vi "ProcAndStates.vi"(0 "spreadsheet string":string=" Инициализация\r\nНачало\r\nВосстановлениеУправления\r\nНачалоРаботы\r\n ОстановВсехПроцессовИстартПроцИнициализация\r\nНачало\r\n КонтрольДостоверности\r\nНачало\r\nОстановПроцессов\r\nСообК_ГУИ_НЕТ_ДОСТОВЕРНОСТИ\r\nНарушениеСвязи\r\n КонтрольДостоверностиОткрытияЗатвораВакуумного\r\nНачало\r\nСменаСостоянияВКЛ\r\nСменаСостоянияВЫКЛ\r\nТрафикПауза\r\nНарушениеСвязи\r\n КонтрольДостоверностиОткрЗатВакуумного\r\nНачало\r\nСообК_ГУИ_ЕСТЬ_ДОСТОВЕРНОСТЬ\r\nОжиданиеНедостоверности\r\nСообК_ГУИ_НЕТ_ДОСТОВЕРНОСТИ\r\nОжиданиеЕстьДостоверность\r\nНарушениеСвязи\r\n КонтрольДостоверностиЗакрЗатВакуумного\r\nНачало\r\nСообК_ГУИ_ЕСТЬ_ДОСТОВЕРНОСТЬ\r\nОжиданиеНедостоверности\r\nСообК_ГУИ_НЕТ_ДОСТОВЕРНОСТИ\r\nОжиданиеЕстьДостоверность\r\nНарушениеСвязи\r\n КонтрольДостоверностиСостоянияСапуна\r\nНачало\r\nСообК_ГУИ_ЕСТЬ_ДОСТОВЕРНОСТЬ\r\nОжиданиеНедостоверности\r\nСообК_ГУИ_НЕТ_ДОСТОВЕРНОСТИ\r\nОжиданиеЕстьДостоверность\r\nНарушениеСвязи\r\n КонтрольДостоверностиСостоянияУстройстваПлавПуска\r\nНачало\r\nСообК_ГУИ_ЕСТЬ_ДОСТОВЕРНОСТЬ\r\nОжиданиеНедостоверности\r\nСообК_ГУИ_НЕТ_ДОСТОВЕРНОСТИ\r\nОжиданиеЕстьДостоверность\r\nНарушениеСвязи\r\n КонтрольДостоверностиСостоянияПитанияВакуумногоНасоса\r\nНачало\r\nСообК_ГУИ_ЕСТЬ_ДОСТОВЕРНОСТЬ\r\nОжиданиеНедостоверности\r\nСообК_ГУИ_НЕТ_ДОСТОВЕРНОСТИ\r\nОжиданиеЕстьДостоверность\r\nНарушениеСвязи\r\n КонтрольДостоверностиСостоянияПитанияВентилятора\r\nНачало\r\nСообК_ГУИ_ЕСТЬ_ДОСТОВЕРНОСТЬ\r\nОжиданиеНедостоверности\r\nСообК_ГУИ_НЕТ_ДОСТОВЕРНОСТИ\r\nОжиданиеЕстьДостоверность\r\nНарушениеСвязи\r\n КонтрольДостоверностиСостоянияПитанияРегТемпературы\r\nНачало\r\nСообК_ГУИ_ЕСТЬ_ДОСТОВЕРНОСТЬ\r\nОжиданиеНедостоверности\r\nСообК_ГУИ_НЕТ_ДОСТОВЕРНОСТИ\r\nОжиданиеЕстьДостоверность\r\nНарушениеСвязи\r\n КонтрольДостоверностиСостоянияПитанияРегУровня\r\nНачало\r\nСообК_ГУИ_ЕСТЬ_ДОСТОВЕРНОСТЬ\r\nОжиданиеНедостоверности\r\nСообК_ГУИ_НЕТ_ДОСТОВЕРНОСТИ\r\nОжиданиеЕстьДостоверность\r\nНарушениеСвязи\r\n КонтрольДостоверностиУровняВодыМинимум\r\nНачало\r\nСообК_ГУИ_ЕСТЬ_ДОСТОВЕРНОСТЬ\r\nОжиданиеНедостоверности\r\nСообК_ГУИ_НЕТ_ДОСТОВЕРНОСТИ\r\nОжиданиеЕстьДостоверность\r\nНарушениеСвязи\r\n КонтрольДостоверностиУровняВодыМаксимум\r\nНачало\r\nСообК_ГУИ_ЕСТЬ_ДОСТОВЕРНОСТЬ\r\nОжиданиеНедостоверности\r\nСообК_ГУИ_НЕТ_ДОСТОВЕРНОСТИ\r\nОжиданиеЕстьДостоверность\r\nНарушениеСвязи\r\n КонтрольДостоверностиСостоянияПитанияНасОхлаждения\r\nНачало\r\nСообК_ГУИ_ЕСТЬ_ДОСТОВЕРНОСТЬ\r\nОжиданиеНедостоверности\r\nСообК_ГУИ_НЕТ_ДОСТОВЕРНОСТИ\r\nОжиданиеЕстьДостоверность\r\nНарушениеСвязи\r\n ЧтениеФактПараметров_с_Датчиков\r\nНачало\r\n РЕГУЛЯТОР_ТРАФИКА\r\nНачало\r\n ЧтениеКольцевогоБуфера\r\nНачало\r\nКонтрольВыполненияК\r\nКонтрольИзмененияНП\r\nНекорректноеСобытие\r\nНарушениеСвязи\r\n ОбработкаКомандИзмененияНП_от_ГУИ\r\nАнализ\r\nПодтверждениеИзмененияНП\r\nНекорректноеСобытие\r\nНарушениеСвязи\r\n ОбработкаКомандУправления_от_ГУИ\r\nАнализ\r\nНекорректноеСобытие\r\nПередачаСообщенияСПараметромГУИ\r\nНарушениеСвязи\r\n КонтрольИзменения_ФП_P_ВбакеКомпрессора\r\nНачало\r\nКонтрольИзменения\r\nСообщОбИзменении\r\nТрафикПауза\r\nНарушениеСвязи\r\n КонтрольИзменения_ФП_P_Впатрубке\r\nНачало\r\nКонтрольИзменения\r\nСообщОбИзменении\r\nТрафикПауза\r\nНарушениеСвязи\r\n КонтрольИзменения_ФП_T_Врубашке\r\nНачало\r\nКонтрольИзменения\r\nСообщОбИзменении\r\nТрафикПауза\r\nНарушениеСвязи\r\n КонтрольИзменения_ФП_T_Вбаке\r\nНачало\r\nКонтрольИзменения\r\nСообщОбИзменении\r\nТрафикПауза\r\nНарушениеСвязи\r\n КонтрольИзменения_ФП_P_ВтрубеСидер\r\nНачало\r\nКонтрольИзменения\r\nСообщОбИзменении\r\nТрафикПауза\r\nНарушениеСвязи\r\n КонтрольВеличиныОткачкиВауумнойТрубыСидеростата\r\nНачало\r\nАнализОткачки\r\n КонтрольГотовностиВакуума_в_Вакуумной_Трубе\r\nНачало\r\nДавлениеНормальное\r\nДавлениеВысокое\r\nЗадержка\r\nНарушениеСвязи\r\n КонтрольУровняВодыБакаОхлаждения\r\nНачало\r\nНизкийУровеньВоды\r\nВысокийУровеньВоды\r\nУровеньВодыВнорме\r\nЗадержка\r\nНарушениеСвязи\r\n КонтрольТемпературыВодыБакаОхлаждения\r\nНачало\r\nНизкаяТемператураВоды\r\nВысокаяТемператураВоды\r\nТемператураВнорме\r\nЗадержка\r\nНарушениеСвязи\r\n КонтрольТемпературыРубашкиОхлаждения\r\nНачало\r\nНизкаяТемператураВоды\r\nВысокаяТемператураВоды\r\nТемператураВнорме\r\nЗадержка\r\nНарушениеСвязи\r\n КонтрольДавленияВбакеКомпрессора\r\nНачало\r\nНизкоеДавление\r\nДавлениеВнорме\r\nЗадержка\r\nНарушениеСвязи\r\n ВКЛ_ПИТ_ВЕНТИЛЯТОР\r\nНачало\r\nКонтрольВключения\r\nПередачаСообщения\r\nОшибка\r\nНарушениеСвязи\r\n ВЫК_ПИТ_ВЕНТИЛЯТОР\r\nНачало\r\nКонтрольВыключения\r\nПередачаСообщения\r\nОшибка\r\nНарушениеСвязи\r\n КонтрольСостоянияПитанияВентилятора\r\nНачало\r\nСменаСостоянияВКЛ\r\nСменаСостоянияВЫКЛ\r\nНарушениеСвязи\r\n КонтрольСпонтанногоВыключенияВентилятора\r\nКонтроль\r\nОшибка\r\nНарушениеСвязи\r\n КонтрольСпонтанногоВключенияВентилятора\r\nКонтроль\r\nОшибка\r\nНарушениеСвязи\r\n КонтрольСостоянияЗатвораВакуумного\r\nНачало\r\nСменаСостоянияСреднего\r\nСменаСостоянияЗакрытия\r\nСменаСостоянияОткрытия\r\nСменаСостоянияОшибки\r\nНарушениеСвязи\r\n ОТКР_ЗАТВОР_ВАК\r\nНачало\r\nКонтроль\r\nПередачаСообщения\r\nОшибка\r\nНарушениеСвязи\r\n ЗАКР_ЗАТВОР_ВАК\r\nНачало\r\nКонтроль\r\nПередачаСообщения\r\nОшибка\r\nНарушениеСвязи\r\n КонтрольСпонтанногоЗакрытияЗатвораВакуумного\r\nКонтрольЗакрытия\r\nОшибка\r\nНарушениеСвязи\r\n КонтрольСпонтанногоОткрытияЗатвораВакуумного\r\nКонтроль\r\nОшибка\r\nНарушениеСвязи\r\n ОТКР_САПУН\r\nНачало\r\nКонтрольОткрытия\r\nПередачаСообщения\r\nОшибка\r\nНарушениеСвязи\r\n ЗАКР_САПУН\r\nНачало\r\nКонтрольЗакрытия\r\nПередачаСообщения\r\nОшибка\r\nНарушениеСвязи\r\n КонтрольСостоянияПитанияСапуна\r\nНачало\r\nСменаСостоянияВКЛ\r\nСменаСостоянияВЫКЛ\r\nНарушениеСвязи\r\n КонтрольСпонтанногоЗакрытияСапуна\r\nКонтрольЗакрытия\r\nОшибка\r\nНарушениеСвязи\r\n КонтрольСпонтанногоОткрытияСапуна\r\nКонтроль\r\nОшибка\r\nНарушениеСвязи\r\n ВКЛ_ПИТ_ВАК_НАСОСА\r\nНачало\r\nКонтрольВключения\r\nПередачаСообщения\r\nОшибка\r\nНарушениеСвязи\r\n ВЫК_ПИТ_ВАК_НАСОСА\r\nНачало\r\nКонтрольВыключения\r\nОшибка\r\nНарушениеСвязи\r\nПередачаСообщения\r\n КонтрольСостоянияПитанияВакуумногоНасоса\r\nНачало\r\nСменаСостоянияВКЛ\r\nСменаСостоянияВЫКЛ\r\nНарушениеСвязи\r\n КонтрольСпонтанногоВыключенияВакНасоса\r\nКонтроль\r\nОшибка\r\nНарушениеСвязи\r\n КонтрольСпонтанногоВключенияВакНасоса\r\nКонтроль\r\nОшибка\r\nНарушениеСвязи\r\n ВКЛ_ПИТ_РЕГ_Т\r\nНачало\r\nКонтрольВключения\r\nПередачаСообщения\r\nОшибка\r\nНарушениеСвязи\r\n ВЫК_ПИТ_РЕГ_Т\r\nНачало\r\nКонтрольВыключения\r\nПередачаСообщения\r\nОшибка\r\nНарушениеСвязи\r\n КонтрольСостоянияПитанияРЕГ_Т\r\nНачало\r\nСменаСостоянияВКЛ\r\nСменаСостоянияВЫКЛ\r\nНарушениеСвязи\r\n КонтрольСпонтанногоВыключенияРЕГ_Т\r\nКонтроль\r\nОшибка\r\nНарушениеСвязи\r\n КонтрольСпонтанногоВключенияРЕГ_Т\r\nКонтроль\r\nОшибка\r\nНарушениеСвязи\r\n ВКЛ_ПИТ_РЕГ_УР\r\nНачало\r\nКонтроль\r\nПередачаСообщения\r\nОшибка\r\nНарушениеСвязи\r\n ВЫК_ПИТ_РЕГ_УР\r\nНачало\r\nКонтроль\r\nПередачаСообщения\r\nОшибка\r\nНарушениеСвязи\r\n КонтрольСостоянияПитанияРЕГ_УР\r\nНачало\r\nСменаСостоянияВКЛ\r\nСменаСостоянияВЫКЛ\r\nНарушениеСвязи\r\n КонтрольСпонтанногоВыключенияРЕГ_УР\r\nКонтроль\r\nОшибка\r\nНарушениеСвязи\r\n КонтрольСпонтанногоВключенияРЕГ_УР\r\nКонтроль\r\nОшибка\r\nНарушениеСвязи\r\n ВКЛ_ПИТ_НАС_ОХЛ\r\nНачало\r\nВключениеПитания\r\nКонтроль\r\nПередачаСообщения\r\nОшибка\r\nНарушениеСвязи\r\n ВЫК_ПИТ_НАС_ОХЛ\r\nНачало\r\nКонтроль\r\nПередачаСообщения\r\nОшибка\r\nНарушениеСвязи\r\n КонтрольСостоянияПитанияНАС_ОХЛ\r\nНачало\r\nСменаСостоянияВКЛ\r\nСменаСостоянияВЫКЛ\r\nНарушениеСвязи\r\n КонтрольСпонтанногоВыключенияНасосаОхлаждения\r\nКонтроль\r\nОшибка\r\nНарушениеСвязи\r\n КонтрольСпонтанногоВключенияНасосаОхлаждения\r\nКонтроль\r\nОшибка\r\nНарушениеСвязи\r\n ВКЛ_УСТР_ПЛАВ_ПУСКА\r\nНачало\r\nКонтроль\r\nПередачаСообщения\r\nОшибка\r\nНарушениеСвязи\r\n ВЫК_УСТР_ПЛАВ_ПУСКА\r\nНачало\r\nКонтрольВыключения\r\nПередачаСообщения\r\nОшибка\r\nНарушениеСвязи\r\n КонтрольСостоянияПитанияПЛАВ_ПУСКА\r\nНачало\r\nСменаСостоянияВКЛ\r\nСменаСостоянияВЫКЛ\r\nНарушениеСвязи\r\n КонтрольСпонтанногоВыключенияПлавнПуска\r\nКонтроль\r\nОшибка\r\nНарушениеСвязи\r\n КонтрольСпонтанногоВключенияПлавнПуска\r\nКонтроль\r\nОшибка\r\nНарушениеСвязи\r\n ВКЛ_ВАКУУМИРОВАНИЕ_ТРУБЫ\r\nНачало\r\nПроверкаНеобходимостиВакуумирования\r\nПередачаСообщения\r\nКонтрольВключенияВакПодсистемы\r\nЗапоминаемДавлениеВвакуумнойТрубе\r\nКонтрольТемпературыРубашки\r\nКонтрольРаботыОборудования\r\nКонтрольДавления\r\nСообщениеОКонцеВакуумирования\r\nПаузаНаРазвакуумированиеТрубы\r\nПаузаНаОткачкуВвакуумнойТрубе\r\nПроверкаУменьшенияДавленияВпатрубке\r\nОткачкаОтсутствует\r\nВыключениеВакуумнойПодсистемы\r\nСообщениеОбОтказеВакуумирования\r\nНарушениеСвязи\r\n ВЫК_ВАКУУМИРОВАНИЕ_ТРУБЫ\r\nНачало\r\nПередачаСообщения\r\nВыключениеВакуумнойПодсистемы\r\nНарушениеСвязи\r\n ВКЛ_ВАКУУМНУЮ_ПОДСИСТЕМУ\r\nНачало\r\nВключениеПитанияРегУровня\r\nКонтрольВключенияПитРегУр\r\nКонтрольГотовностиУровняВодыБО\r\nВключениеРегТ\r\nКонтрольВключенияРегТ\r\nКонтрольПревышенияТемпературыВодыБО\r\nКонтрольГотовностиТемпературыВодыБО\r\nВключаемВентилятор\r\nКонтрольВключенияВентилятора\r\nКонтрольВключенияПитанияНасосаОхлаждения\r\nКонтрольЗакрытияЗатвораВакуумного\r\nКонтрольОткрытияСапуна\r\nКонтрольТемпературыРубашки\r\nПодачаПитанияНаВакуумныйНасос\r\nКонтрольПитанияВакуумногоНасоса\r\nВключениеУстройстваПлавногоПуска\r\nКонтрольВлюченияПлавногоПуска\r\nТаймаутПередЗакрытиемСапуна\r\nЗакрытиеСапуна\r\nКонтрольЗакрытияСапуна\r\nЗапоминаемДавлениеВпатрубке\r\nКонтрольДавления\r\nПаузаНаОткачкуВпатрубке\r\nПроверкаУменьшенияДавленияВпатрубке\r\nКонтрольОткрытияЗВ\r\nОшибка\r\nВыключениеПоОшибке\r\nСообщениеОбОтказеВакуумирования\r\nНарушениеСвязи\r\n ВЫК_ВАКУУМНУЮ_ПОДСИСТЕМУ\r\nНачало\r\nКонтрольЗакрытияЗатвораВакуумного\r\nКонтрольОткрытияСапуна\r\nТаймаутПередВыключениемПитанияВакуумногоНасоса\r\nВыключаемУППВакуумногоНасоса\r\nКонтрольВыключенияПитанияУППВакуумногоНасоса\r\nКонтрольВыключенияПитанияВакуумногоНасоса\r\nКонтрольВыключенияНасосаОхлаждения\r\nКонтрольВыключенияВентилятора\r\nСообщениеОбОтказеВыклВакСистемы\r\nНарушениеСвязи\r\n") -> (1 "PROCESSES":string[](array[string])=["Инициализация", "ОстановВсехПроцессовИстартПроцИнициализация", "КонтрольДостоверности", "КонтрольДостоверностиОткрытияЗатвораВакуумного", "КонтрольДостоверностиОткрЗатВакуумного", "КонтрольДостоверностиЗакрЗатВакуумного", "КонтрольДостоверностиСостоянияСапуна", "КонтрольДостоверностиСостоянияУстройстваПлавПуска", "КонтрольДостоверностиСостоянияПитанияВакуумногоНасоса", "КонтрольДостоверностиСостоянияПитанияВентилятора", "КонтрольДостоверностиСостоянияПитанияРегТемпературы", "КонтрольДостоверностиСостоянияПитанияРегУровня", "КонтрольДостоверностиУровняВодыМинимум", "КонтрольДостоверностиУровняВодыМаксимум", "КонтрольДостоверностиСостоянияПитанияНасОхлаждения", "ЧтениеФактПараметров_с_Датчиков", "РЕГУЛЯТОР_ТРАФИКА", "ЧтениеКольцевогоБуфера", "ОбработкаКомандИзмененияНП_от_ГУИ", "ОбработкаКомандУправления_от_ГУИ", "КонтрольИзменения_ФП_P_ВбакеКомпрессора", "КонтрольИзменения_ФП_P_Впатрубке", "КонтрольИзменения_ФП_T_Врубашке", "КонтрольИзменения_ФП_T_Вбаке", "КонтрольИзменения_ФП_P_ВтрубеСидер", "КонтрольВеличиныОткачкиВауумнойТрубыСидеростата", "КонтрольГотовностиВакуума_в_Вакуумной_Трубе", "КонтрольУровняВодыБакаОхлаждения", "КонтрольТемпературыВодыБакаОхлаждения", "КонтрольТемпературыРубашкиОхлаждения", "КонтрольДавленияВбакеКомпрессора", "ВКЛ_ПИТ_ВЕНТИЛЯТОР", "ВЫК_ПИТ_ВЕНТИЛЯТОР", "КонтрольСостоянияПитанияВентилятора", "КонтрольСпонтанногоВыключенияВентилятора", "КонтрольСпонтанногоВключенияВентилятора", "КонтрольСостоянияЗатвораВакуумного", "ОТКР_ЗАТВОР_ВАК", "ЗАКР_ЗАТВОР_ВАК", "КонтрольСпонтанногоЗакрытияЗатвораВакуумного", "КонтрольСпонтанногоОткрытияЗатвораВакуумного", "ОТКР_САПУН", "ЗАКР_САПУН", "КонтрольСостоянияПитанияСапуна", "КонтрольСпонтанногоЗакрытияСапуна", "КонтрольСпонтанногоОткрытияСапуна", "ВКЛ_ПИТ_ВАК_НАСОСА", "ВЫК_ПИТ_ВАК_НАСОСА", "КонтрольСостоянияПитанияВакуумногоНасоса", "КонтрольСпонтанногоВыключенияВакНасоса", "КонтрольСпонтанногоВключенияВакНасоса", "ВКЛ_ПИТ_РЕГ_Т", "ВЫК_ПИТ_РЕГ_Т", "КонтрольСостоянияПитанияРЕГ_Т", "КонтрольСпонтанногоВыключенияРЕГ_Т", "КонтрольСпонтанногоВключенияРЕГ_Т", "ВКЛ_ПИТ_РЕГ_УР", "ВЫК_ПИТ_РЕГ_УР", "КонтрольСостоянияПитанияРЕГ_УР", "КонтрольСпонтанногоВыключенияРЕГ_УР", "КонтрольСпонтанногоВключенияРЕГ_УР", "ВКЛ_ПИТ_НАС_ОХЛ", "ВЫК_ПИТ_НАС_ОХЛ", "КонтрольСостоянияПитанияНАС_ОХЛ", "КонтрольСпонтанногоВыключенияНасосаОхлаждения", "КонтрольСпонтанногоВключенияНасосаОхлаждения", "ВКЛ_УСТР_ПЛАВ_ПУСКА", "ВЫК_УСТР_ПЛАВ_ПУСКА", "КонтрольСостоянияПитанияПЛАВ_ПУСКА", "КонтрольСпонтанногоВыключенияПлавнПуска", "КонтрольСпонтанногоВключенияПлавнПуска", "ВКЛ_ВАКУУМИРОВАНИЕ_ТРУБЫ", "ВЫК_ВАКУУМИРОВАНИЕ_ТРУБЫ", "ВКЛ_ВАКУУМНУЮ_ПОДСИСТЕМУ", "ВЫК_ВАКУУМНУЮ_ПОДСИСТЕМУ"], 2 "STATES":string[][](array[string]))   [LabVIEW 2010]
panel:
  out "size(s)":i32[](array[numeric])=[75, 0]
  out "Array":string[](array[string])=["Начало", "КонтрольЗакрытияЗатвораВакуумного", "КонтрольОткрытияСапуна", "ТаймаутПередВыключениемПитанияВакуумногоНасоса", "ВыключаемУППВакуумногоНасоса", "КонтрольВыключенияПитанияУППВакуумногоНасоса", "КонтрольВыключенияПитанияВакуумногоНасоса", "КонтрольВыключенияНасосаОхлаждения", "КонтрольВыключенияВентилятора", "СообщениеОбОтказеВыклВакСистемы", "НарушениеСвязи"]
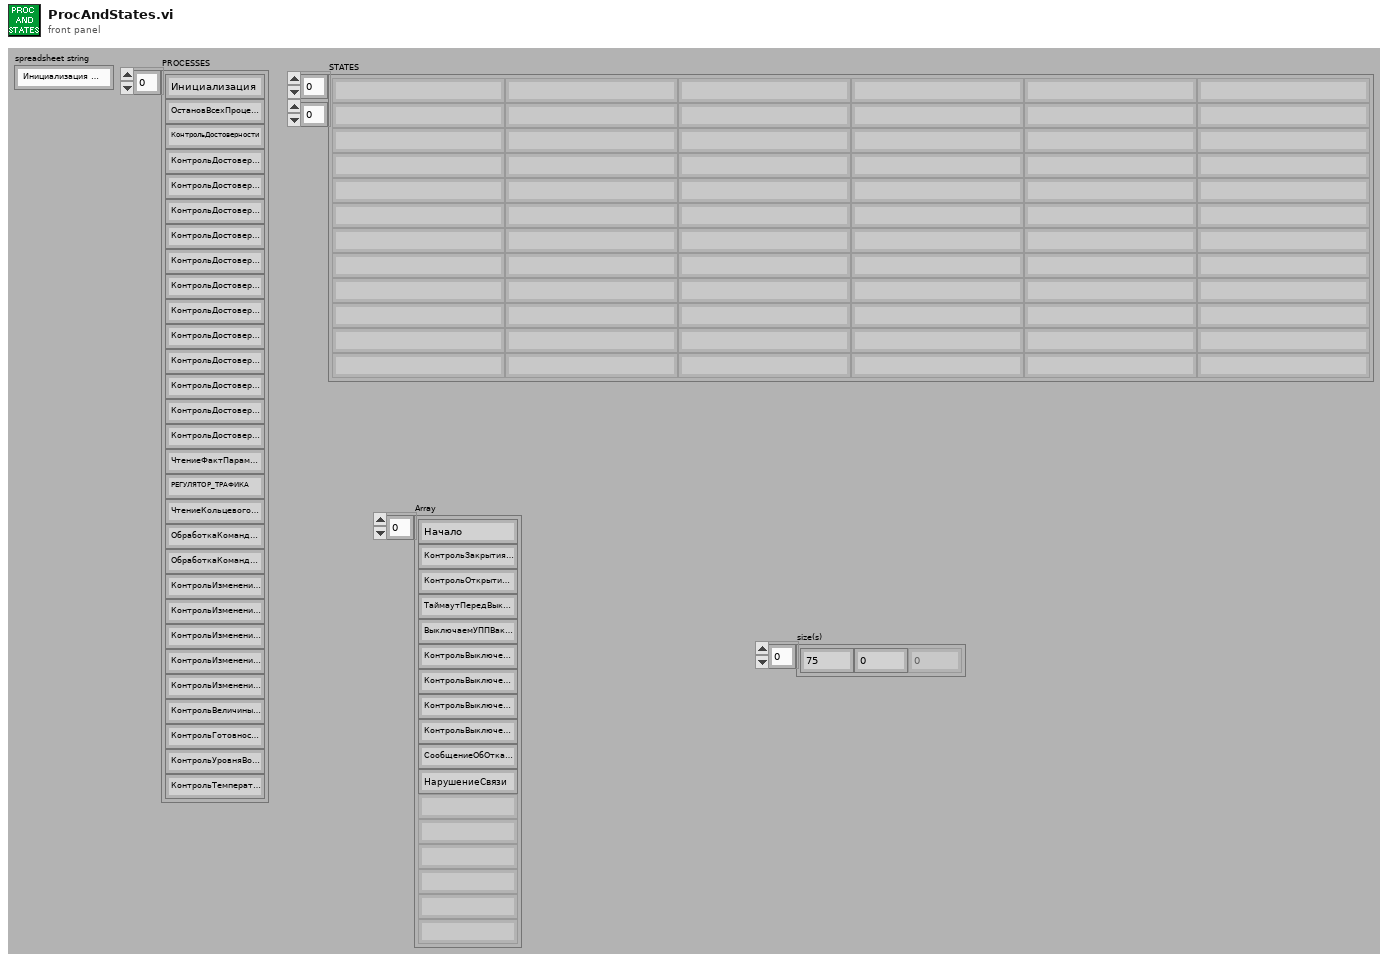
[diagram p1: front panel]
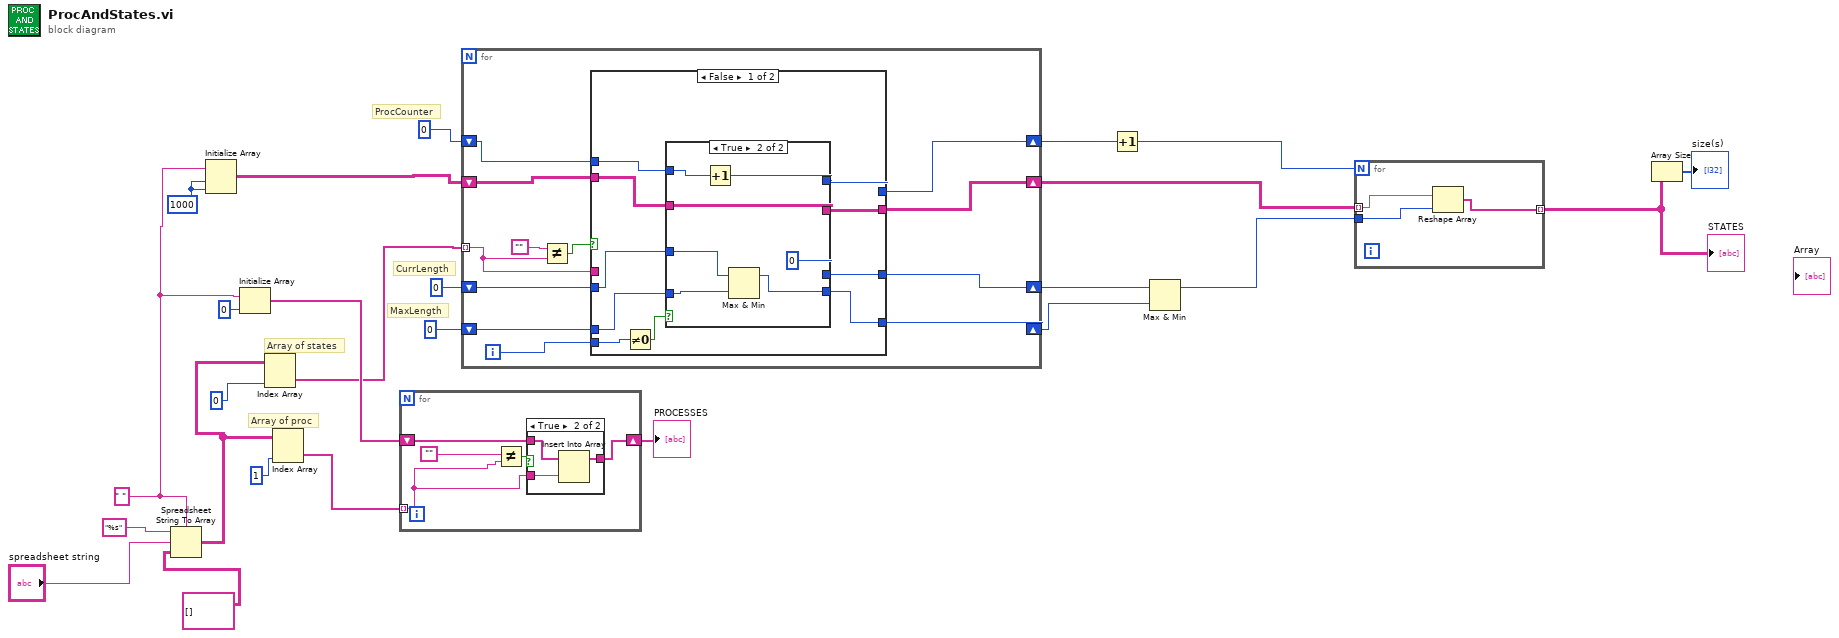
[diagram p0: block diagram]
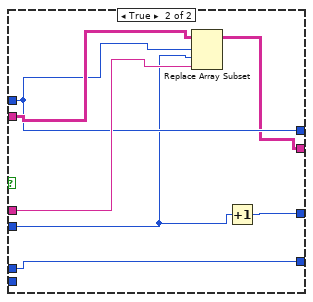
[diagram p3: hidden frame]
diagram:
  w9 = 1000 ("dimension size")
  w10 = " " ("delimiter (Tab)")
  # "CurrLength"
  # "MaxLength"
  # "ProcCounter"
  # "Array of proc"
  # "Array of states"
  n1 = Spreadsheet String To Array(delimiter (Tab)=w10, format string="%s", spreadsheet string="spreadsheet string", array type (2D Dbl)=string[][] []) -> (array=w24:string[][])
  n2 = Initialize Array(w10, w9, w9) -> (w14:string[][])
  n3 = Initialize Array(w10, 0 ("dimension size")) -> (w20:string[])
  n4 = Index Array(array=w24, index (col)=0 ("index (row)")) -> (element=w11:string[])  [unwired: 1 in]
  n5 = Index Array(array=w24, index (col)=1 ("index (row)")) -> (element=w18:string[])  [unwired: 1 in]
  n6 = for {
    tunnel: w18 -> [w29] mode=indexing
    shift-right: [w27] -> w19
    shift-left: w20 -> [w28]
    n7 = Not Equal?(x="", y=w29) -> (x != y?=w30:bool)
    n8 = case shown="True" w30 {
      tunnel: w29 -> [_ w33]
      tunnel: w28 -> [w31 w34]
      tunnel: [w31 w32] -> w27
      frame False {
      }
      frame True {
        n9 = Insert Into Array(array=w34, new element=w33) -> (w32:string[])  [unwired: 1 in]
      }
    }
  }
  "PROCESSES" <- w19
  n10 = for {
    tunnel: w11 -> [w44] mode=indexing
    shift-right: [w40] -> w6
    shift-left: w14 -> [w45]
    shift-right: [w42] -> w5
    shift-left: 0 ("dimension size") -> [w43]
    shift-right: [w39] -> w2
    shift-left: 0 ("dimension size") -> [w41]
    shift-right: [w35] -> w3
    shift-left: 0 ("dimension size") -> [w36]
    i -> [w37]
    n11 = Not Equal?(x="", y=w44) -> (x != y?=w46:bool)
    n12 = case shown="False" w46 {
      tunnel: [w55 w69] -> w40
      tunnel: w45 -> [w56 w73]
      tunnel: w44 -> [_ w72]
      tunnel: w43 -> [w54 w71]
      tunnel: [w47 w71] -> w42
      tunnel: w41 -> [w53 w74]
      tunnel: [w52 w74] -> w39
      tunnel: w37 -> [w51 _]
      tunnel: w36 -> [w49 w68]
      tunnel: [w48 w70] -> w35
      frame False {
        n13 = Not Equal To 0?(x=w51) -> (x != 0?=w50:bool)
        n14 = case shown="True" w50 {
          tunnel: w56 -> [w60 w63]
          tunnel: [w60 w63] -> w55
          tunnel: w54 -> [w58 w67]
          tunnel: [w58 w62] -> w47
          tunnel: w53 -> [w59 w66]
          tunnel: [w59 w61] -> w52
          tunnel: w49 -> [w57 w65]
          tunnel: [w57 0] -> w48
          frame False {
          }
          frame True {
            n15 = Increment(x=w67) -> (x+1=w62:i32)
            n16 = Max & Min(x=w65, y=w66) -> (max(x,y)=w61:i32)  [unwired: 1 out]
          }
        }
      }
      frame True {
        n17 = Replace Array Subset(array=w73, new element=w72, index (row)=w71, index (col)=w68) -> (w69:string[][])
        n18 = Increment(x=w68) -> (x+1=w70:i32)
      }
    }
  }
  n19 = Increment(x=w5) -> (x+1=w4:i32)
  n20 = Max & Min(x=w3, y=w2) -> (max(x,y)=w1:i32)  [unwired: 1 out]
  n21 = for {
    N: w4 -> [_]
    tunnel: w6 -> [w77] mode=indexing
    tunnel: w1 -> [w76]
    tunnel: [w75] -> w8 mode=indexing
    n22 = Reshape Array(w77, w76) -> (w75:string[])
  }
  "STATES" <- w8
  n23 = Array Size(array=w8) -> (size(s)=→"size(s)":i32[])
